vi "Find Port.vi"(9 "Multimetro":T1, 10 "Ports Found":string[](array[string])) -> (2 "Addr Ports":string[](array[string]))   [LabVIEW 2015]
uses:
  controls/Instruments.ctl
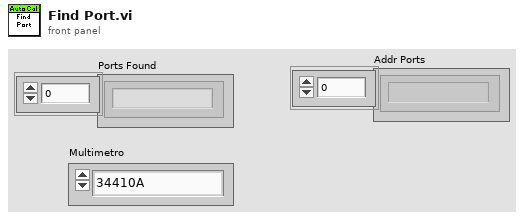
[diagram p1: front panel]
types:
  T1 = typedef "Instruments.ctl" = enum16{"34410A", "34401A", "U1252B", "U1252A", "U1213A", "8845A", "8846A", "189", "289", "DMM4050", "TY720"}
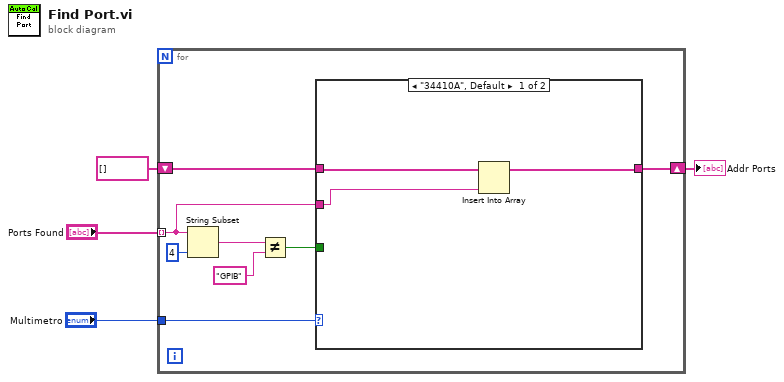
[diagram p0: block diagram]
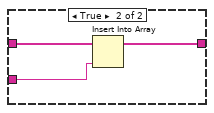
[diagram p3: hidden frame]
diagram:
  n1 = for {
    tunnel: "Ports Found" -> [w7] mode=indexing
    tunnel: "Multimetro" -> [w9]
    shift-right: [w5] -> w1
    shift-left: string[] [] -> [w6]
    n2 = String Subset(string=w7, length (rest)=4 ("length (rest)")) -> (substring=w11:string)  [unwired: 1 in]
    n3 = Not Equal?(x=w11, y="GPIB") -> (x != y?=w8:bool)
    n4 = case shown="\"34410A\", Default" w9 {
      tunnel: w8 -> [_ w19]
      tunnel: w7 -> [w14 w18]
      tunnel: w6 -> [w15 w17]
      tunnel: [w13 w16] -> w5
      frame "34410A", Default {
        n5 = Insert Into Array(array=w15, new element=w14) -> (w13:string[])  [unwired: 1 in]
      }
      frame "U1252B".."U1213A", "189", "289", "TY720" {
        n6 = case shown="False" w19 {
          tunnel: w18 -> [_ w23]
          tunnel: w17 -> [w20 w22]
          tunnel: [w20 w21] -> w16
          frame False {
          }
          frame True {
            n7 = Insert Into Array(array=w22, new element=w23) -> (w21:string[])  [unwired: 1 in]
          }
        }
      }
    }
  }
  "Addr Ports" <- w1
